vi "Configure.vi"(8 "error in":errorcluster, 10 "name":string, 11 "PAS in":refnum<class "PAS.lvclass">) -> (0 "error out":errorcluster, 3 "PAS out":refnum<class "PAS.lvclass">)   [LabVIEW 2016, in "PAS Library.lvlib" / "PAS.lvclass"]
doc: "Configure the instrument class. If there is no config file specified, an error"
uses:
  PAS.lvclass
  G:/sw_repo/For Builds/Reusable/Instrument/Instrument.lvclass
  Data/Main/PAS Data.lvclass
  G:/sw_repo/For Builds/Reusable/Data/Data.lvclass
  Instrument/Instrument.lvclass/Instrument.ctl
  Data/Data.lvclass/Data.ctl
  Commands/Change Speaker Cycle Params/Change Speaker Cycle Params.lvclass
  G:/sw_repo/For Builds/Reusable/Command/Command.lvclass
  Session APIs/File Access/Config Data/Config Data.lvclass/Config Data.ctl
  Commands/Change Speaker Cycle Params/Change Speaker Cycle Params.lvclass/Change Speaker Cycle Params.ctl
  Data/Cell/PAS Cell Data.lvclass/PAS Cell Data.ctl
  PAS.lvclass/PAS.ctl
  Data/Cell/Write Ncell.vi
  Data/Write Data ID.vi
  Data/Cell/Write serializeWF_.vi
  Session APIs/File Access/Config Data/Accessors/Read Ref.vi
  Commands/Change Speaker Cycle Params/Write period.vi
  Commands/Change Speaker Cycle Params/Write length.vi
  Commands/Change Speaker Cycle Params/Write auto_.vi
  Instrument/Read Data.vi
  Instrument/Read Cfg Session.vi
  Instrument/Read ExtCom.vi
  Instrument/Read Log Session.vi
  Instrument/Read CMD.vi
  Instrument/Write Data.vi
  Data/Cell/PAS Cell Data.lvclass
  Read Cells.vi
  Data/Main/Read CellData.vi
  Session APIs/File Access/Config Data/Read Array/Read DBL Array.vi
  <vilib>/Utility/config.llb/Read Key (I32).vi
  <vilib>/Utility/config.llb/Read Key (Boolean).vi
  Cell/Write extParams.vi
  Data/Main/Write CellData.vi
  Instrument/Instrument.lvclass
  Data/Data.lvclass
  Cell/PAS Cell.lvclass
  Session APIs/File Access/Config Data/Config Data.lvclass
  Session APIs/_Session Fwk/Session - Root.lvclass
  Command/Command.lvclass
  <vilib>/Utility/config.llb/NI_LVConfig.lvlib
  Session APIs/Session Log/System Log.lvclass
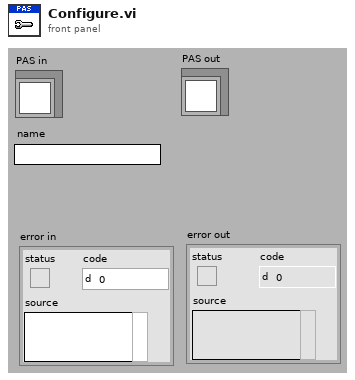
[diagram p1: front panel]
types:
  T1 = typedef "Session - Root.lvclass/Session Handle.ctl" = refnum<data-value>
  T2 = cluster{"tag":string, "section":string, "data":variant}
  T3 = typedef "NI_LVConfig.lvlib/Config Data RefNum.ctl" = refnum<k1>
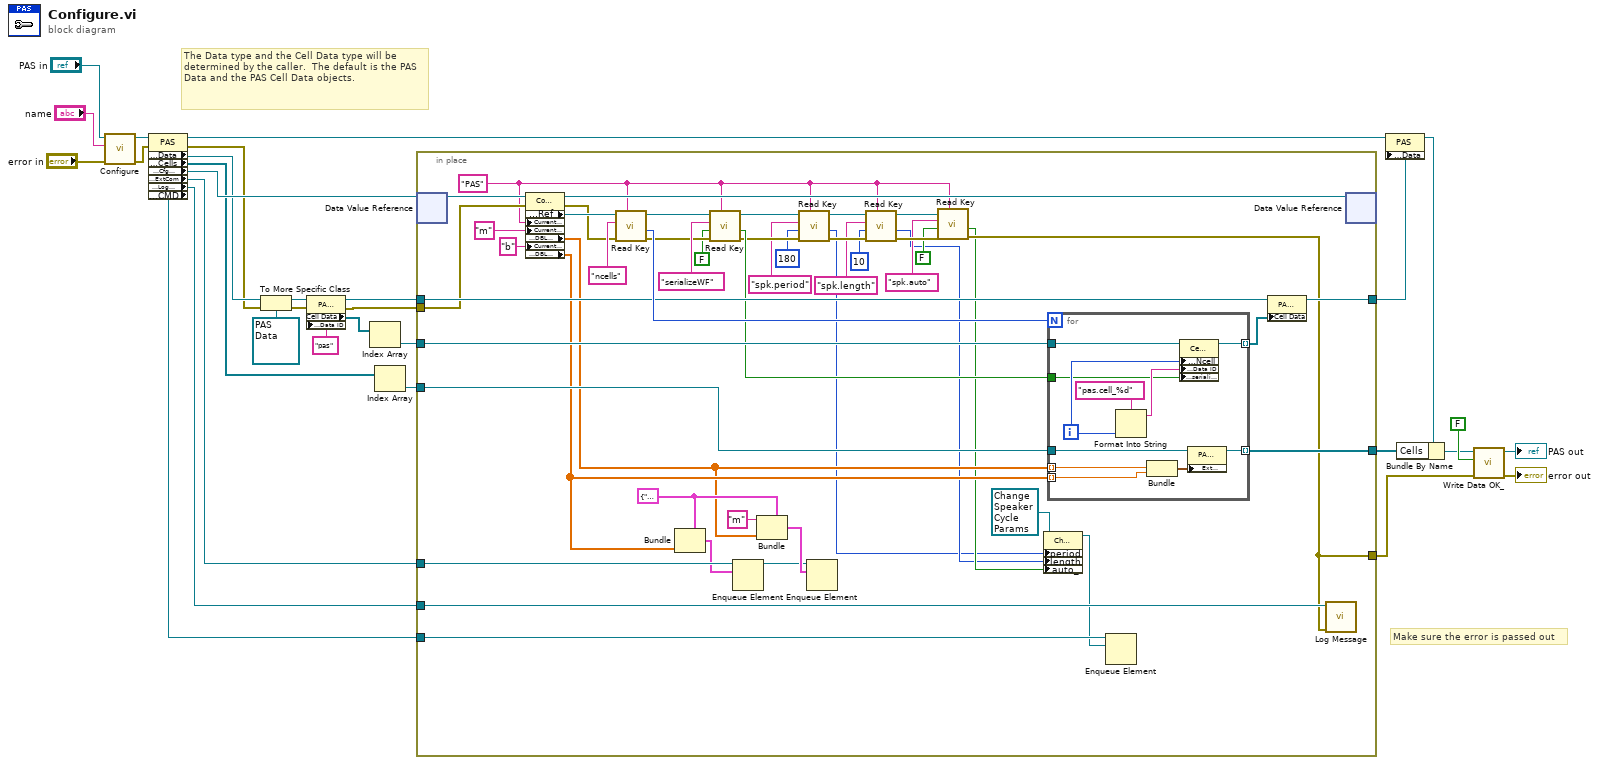
[diagram p0: block diagram]
diagram:
  # "Make sure the error is passed out"
  # "The Data type and the Cell Data type will be determined by the caller.  The default is the PAS Data and the PAS Cell Data objects."
  n1 = call-parent "Configure.vi"("error in"="error in", "name"="name", "Instrument in"="PAS in") -> ("error out"=w26:errorcluster, "Instrument out"=w27:refnum<class "PAS.lvclass">)  [unwired: 7 in]
  n2 = property class="PAS"(reference=w27, error in=w26) -> (reference out=w18:refnum<class "PAS.lvclass">, error out=w6:errorcluster, "Accessors:Data"=w8:refnum<class "Data.lvclass">, "Data Access:Cells"=w11:refnum<class "PAS Cell.lvclass">[], "Accessors:Cfg Session"=w12:refnum<data-value>, "Accessors:ExtCom"=w7:refnum<queue>, "Accessors:Log Session"=w4:T1, "Accessors:CMD"=w1:refnum<queue>)
  n3 = To More Specific Class(target class=refnum<class "PAS Data.lvclass"> refnum ("PAS Data"), reference=w8, error in=w6) -> (specific class reference=w16:refnum<class "PAS Data.lvclass">, error out=w10:errorcluster)
  n4 = property class="PAS Data"(reference=w16, error in=w10, "Accessors:Data ID"="pas" ("Data ID")) -> (reference out=w13:refnum<class "PAS Data.lvclass">, error out=w2:errorcluster, "Cell Data"=w15:refnum<class "PAS Cell Data.lvclass">[])
  n5 = Index Array(array=w15) -> (element=w14:refnum<class "PAS Cell Data.lvclass">)  [unwired: 1 in]
  n6 = Index Array(array=w11) -> (element=w25:refnum<class "PAS Cell.lvclass">)  [unwired: 1 in]
  n7 = in-place {
    in-place-border: w25 -> [w76]
    in-place-border: [w75] -> w24
    in-place-border: [w73] -> w19
    in-place-border: w14 -> [w70]
    in-place-border: w13 -> [w69]
    in-place-border: w7 -> [w60]
    in-place-border: w4 -> [w52]
    in-place-border: [w40] -> w3
    in-place-border: w2 -> [w51]
    in-place-border: w1 -> [w50]
    w58 = T2 {"tag"="b", "section"="pas", "data"=variant} ("element")
    w45 = "PAS" ("section")
    n8 = in-place-dvr #1(w12) -> (w79:refnum<class "Config Data.lvclass">)  [unwired: 1 out]
    n9 = property class="Config Data"(reference=w79, error in=w51, "Current Section"=w45, "Current Key"="m", "Current Key"="b") -> (reference out=w66:refnum<class "Config Data.lvclass">, error out=w71:errorcluster, "Accessors:Ref"=w72:T3, "Read Array Data:DBL Data"=w56:dbl[], "Read Array Data:DBL Data"=w59:dbl[])
    n10 = call-poly <vilib>:"Read Key.vi"("section"=w45, "error in (no error)"=w71, "key"="ncells", "refnum"=w72) -> ("error out"=w63:errorcluster, "value"=w77:i32, "refnum out"=w65:T3)  [unwired: 4 in, 1 out]
    n11 = Bundle(cluster=w58, "data"=w59) -> (w55:T2)  [unwired: 2 in]
    n12 = call-poly <vilib>:"Read Key.vi"("section"=w45, "error in (no error)"=w63, "default value"=FALSE, "key"="serializeWF", "refnum"=w65) -> ("error out"=w43:errorcluster, "value"=w62:bool, "refnum out"=w49:T3)  [unwired: 3 in, 1 out]
    n13 = Enqueue Element(queue=w60, element=w55) -> (queue out=w53:refnum<queue>)  [unwired: 2 in, 2 out]
    n14 = Bundle(cluster=w58, "tag"="m", "data"=w56) -> (w54:T2)  [unwired: 1 in]
    n15 = call-poly <vilib>:"Read Key.vi"("section"=w45, "error in (no error)"=w43, "default value"=180, "key"="spk.period", "refnum"=w49) -> ("error out"=w44:errorcluster, "value"=w32:i32, "refnum out"=w48:T3)  [unwired: 3 in, 1 out]
    n16 = Enqueue Element(queue=w53, element=w54) -> ()  [unwired: 2 in, 3 out]
    n17 = call-poly <vilib>:"Read Key.vi"("section"=w45, "error in (no error)"=w44, "default value"=10, "key"="spk.length", "refnum"=w48) -> ("error out"=w47:errorcluster, "value"=w33:i32, "refnum out"=w46:T3)  [unwired: 3 in, 1 out]
    n18 = call-poly <vilib>:"Read Key.vi"("section"=w45, "error in (no error)"=w47, "default value"=FALSE, "key"="spk.auto", "refnum"=w46) -> ("error out"=w40:errorcluster, "value"=w34:bool)  [unwired: 3 in, 2 out]
    n19 = property class="Change Speaker Cycle Params"(reference=refnum<class "Change Speaker Cycle Params.lvclass"> refnum ("PAS Library.lvlib:Change Speaker Cycle Params"), "period"=w32, "length"=w33, "auto_"=w34) -> (reference out=w31:refnum<class "Change Speaker Cycle Params.lvclass">)  [unwired: 1 in, 1 out]
    n20 = for {
      N: w77 -> [_]
      tunnel: w76 -> [w90]
      tunnel: [w89] -> w75 mode=indexing
      tunnel: [w84] -> w74 mode=indexing
      tunnel: w70 -> [w85]
      tunnel: w56 -> [w88] mode=indexing
      tunnel: w59 -> [w87] mode=indexing
      tunnel: w62 -> [w80]
      i -> [w83]
      n21 = Format Into String(format string="pas.cell_%d", w83) -> (resulting string=w81:string)  [unwired: 2 in, 1 out]
      n22 = Bundle(w88, w87) -> (w86:cluster{dbl, dbl})  [unwired: 1 in]
      n23 = property class="Cell Data"(reference=w85, "Accessors:Ncell"=w83, "Accessors:Data ID"=w81, "Accessors:serializeWF_"=w80) -> (reference out=w84:refnum<class "PAS Cell Data.lvclass">)  [unwired: 1 in, 1 out]
      n24 = property class="PAS Cell"(reference=w90, "Ext Params"=w86) -> (reference out=w89:refnum<class "PAS Cell.lvclass">)  [unwired: 1 in, 1 out]
    }
    n25 = Enqueue Element(queue=w50, element=w31) -> ()  [unwired: 2 in, 3 out]
    n26 = property class="PAS Data"(reference=w69, "Cell Data"=w74) -> (reference out=w73:refnum<class "PAS Data.lvclass">)  [unwired: 1 in, 1 out]
    n27 = call "Log Message.vi"("error in"=w40, "session in"=w52) -> ()  [unwired: 8 in, 2 out]
    n28 = in-place-dvr #1(w66) -> ()  [unwired: 2 out]
  }
  n29 = property class="PAS"(reference=w18, "Accessors:Data"=w19) -> (reference out=w20:refnum<class "PAS.lvclass">)  [unwired: 1 in, 1 out]
  n30 = Bundle By Name(cluster=w20, "Cells"=w24) -> (w21:refnum<class "PAS.lvclass">)
  n31 = call "Write Data OK_.vi"("error in (no error)"=w3, "Data OK?"=FALSE ("goodData"), "Instrument in"=w21) -> ("error out"=→"error out":errorcluster, "Instrument out"=→"PAS out":refnum<class "PAS.lvclass">)  [unwired: 7 in]
